vi "temperature conversion cases.vi"() -> ()   [LabVIEW 2018]
panel:
  in  "Numeric":dbl
  out "Thermometer":dbl(slide) scale=0.0..100.0
  in  "x":dbl
  out "Thermometer F":dbl(slide) scale=0.0..212.0
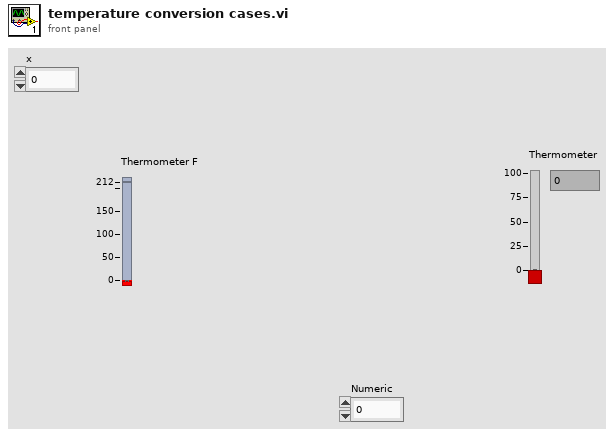
[diagram p1: front panel]
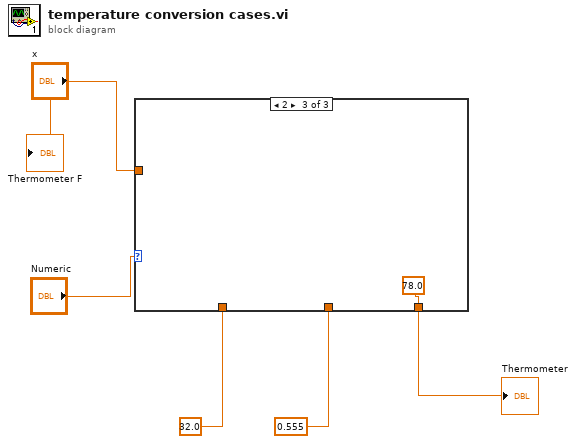
[diagram p0: block diagram]
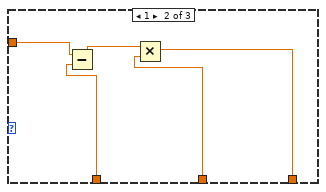
[diagram p3: hidden frame]
diagram:
  n1 = case shown="2" "Numeric" {
    tunnel: 32.0 ("y") -> [_ w10 _]
    tunnel: 0.555 ("y") -> [_ w9 _]
    tunnel: [w6 w7 78.0 ("x")] -> w2
    tunnel: "x" -> [w6 w8 _]
    frame 0, Default {
    }
    frame 1 {
      n2 = Subtract(x=w8, y=w10) -> (x-y=w11:dbl)
      n3 = Multiply(x=w11, y=w9) -> (x*y=w7:dbl)
    }
    frame 2 {
    }
  }
  "Thermometer" <- w2
  "Thermometer F" <- "x"
